vi "NeighborsRegressors.vi"   [LabVIEW 2020]
doc: "Polymorphic VI for neighbors regressors"
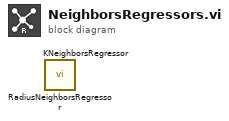
[diagram p0: block diagram]
diagram:
  n1 = call "RadiusNeighborsRegressor.vi"() -> ()  [unwired: 10 in, 2 out]
  n2 = call "KNeighborsRegressor.vi"() -> ()  [unwired: 10 in, 2 out]
